vi "NF LI56xx dvr qDATA DATA.vi"(8 "error in":errorcluster caption="error in (no error)" {"code" format="%.0x"}, 11 "VISA resource name":refnum<visa-resource-name>) -> (0 "error out":errorcluster {"code" format="%.0x"}, 3 "VISA resource name copy":refnum<visa-resource-name>)   [LabVIEW 2019]
doc: "Queries the contents of the measurement data buffer (the measurement values)."
panel:
  out "measurement data":string
  in  "start position":u32 max=65536 step=1
  in  "block length":u32=1 min=1 max=65536 step=1
  in  "set data buffer":enum16{"BUF1", "BUF2", "BUF3"}(ring)=enum."BUF2"
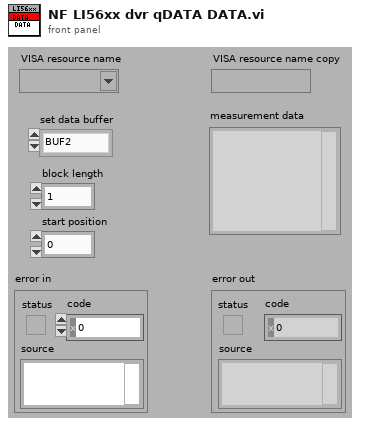
[diagram p1: front panel]
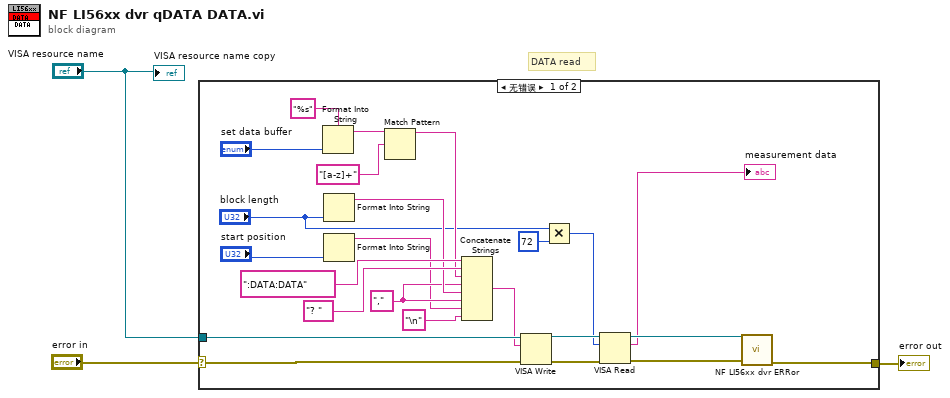
[diagram p0: block diagram]
diagram:
  # "DATA read"
  n1 = case shown="无错误" "error in" {
    selector: "error in" -> [w27 w28]
    tunnel: [w25 w28] -> w3
    tunnel: "VISA resource name" -> [w26 _]
    frame No Error {
      w10 = "," ("Œ`Ž®•¶Žš—ñ")
      n2 = Format Into String(format string="%s", "set data buffer") -> (resulting string=w22:string)  [unwired: 2 in, 1 out]
      n3 = Format Into String("block length") -> (resulting string=w11:string)  [unwired: 3 in, 1 out]
      n4 = Format Into String("start position") -> (resulting string=w6:string)  [unwired: 3 in, 1 out]
      n5 = Match Pattern(string=w22, regular expression="[a-z]+") -> (before substring=w12:string)  [unwired: 1 in, 3 out]
      n6 = Concatenate Strings(":DATA:DATA" ("•¶Žš—ñ"), "? " ("Œ`Ž®•¶Žš—ñ"), w12, w10, w11, w10, w6, "\n" ("Œ`Ž®•¶Žš—ñ")) -> (w24:string)
      n7 = VISA Write(VISA resource name=w26, write buffer=w24, error in (no error)=w27) -> (VISA resource name out=w19:refnum<visa-resource-name>, error out=w17:errorcluster)  [unwired: 1 out]
      n8 = Multiply(x="block length", y=72) -> (x*y=w8:u32)
      n9 = VISA Read(VISA resource name=w19, byte count=w8, error in (no error)=w17) -> (VISA resource name out=w18:refnum<visa-resource-name>, read buffer=→"measurement data":string, error out=w16:errorcluster)  [unwired: 1 out]
      n10 = call "NF LI56xx dvr ERRor.vi"("VISA resource name"=w18, "error in (no error)"=w16) -> ("error out"=w25:errorcluster)  [unwired: 10 in, 3 out]
    }
    frame Error {
    }
  }
  "error out" <- w3
  "VISA resource name copy" <- "VISA resource name"
